vi "Enumerate Default Assert Strategies.vi"(11 "Banana":refnum<class "Banana.lvclass">) -> (1 "Strategies":T1, 3 "Banana":refnum<class "Banana.lvclass">)   [LabVIEW 2021, in "Bananas.lvlib" / "Platano.lvclass"]
uses:
  Platano.lvclass
  Banana/Banana.lvclass
  Assertion Strategies -- cluster.ctl
  AssertTrue/AssertTrue.lvclass
  AssertFalse/AssertFalse.lvclass
  AssertEqualValue/AssertEqualValue.lvclass
  AssertEqualType/AssertEqualType.lvclass
  AssertCompareValue/AssertCompareValue.lvclass
  AssetError/AssertError.lvclass
  AssertAlmostEqual/AssertAlmostEqualValue.lvclass
  Banana/Banana.lvclass/Banana.ctl
  <vilib>/LabVIEW Open Source Project/Data Manipulation/Variant/Variant_EmptyCluster.vi
  <vilib>/LabVIEW Open Source Project/Data Manipulation/TypeDescriptor/TypeDescriptor_SetName.vi
  <vilib>/Utility/GetType.llb/TD_Create Cluster.vi
  BananaPeel/BananaPeel.lvclass
  <vilib>/LabVIEW Open Source Project/Data Manipulation/Variant/OpenVariant.lvlib
  Bananas.lvlib
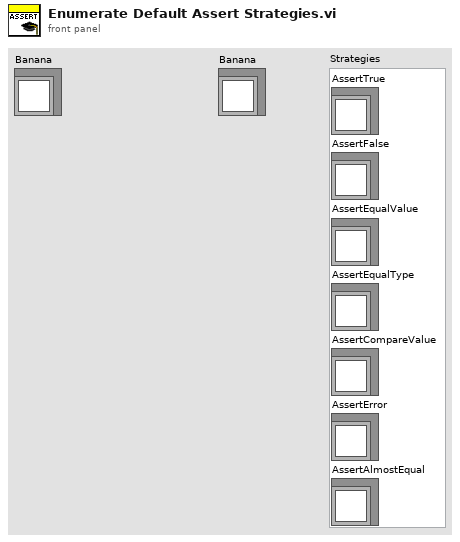
[diagram p1: front panel]
types:
  T1 = typedef "Bananas.lvlib/Assertion Strategies -- cluster.ctl" = cluster{"AssertTrue":refnum<class "AssertTrue.lvclass">, "AssertFalse":refnum<class "AssertFalse.lvclass">, "AssertEqualValue":refnum<class "AssertEqualValue.lvclass">, "AssertEqualType":refnum<class "AssertEqualType.lvclass">, "AssertCompareValue":refnum<class "AssertCompareValue.lvclass">, "AssertError":refnum<class "AssertError.lvclass">, "AssertAlmostEqual":refnum<class "AssertAlmostEqualValue.lvclass">}
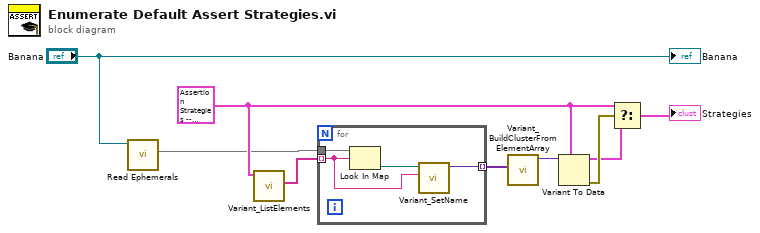
[diagram p0: block diagram]
diagram:
  w3 = T1 {"AssertTrue"=refnum, "AssertFalse"=refnum, "AssertEqualValue"=refnum, "AssertEqualType"=refnum, "AssertCompareValue"=refnum, "AssertError"=refnum, "AssertAlmostEqual"=refnum} ("Strategies")
  n1 = call "Read Ephemerals.vi"("Banana in"="Banana") -> ("Ephemerals"=w1:map{string, refnum<class "BananaPeel.lvclass">})  [unwired: 8 in, 2 out]
  n2 = call <vilib>:"Variant_ListElements.vi"("Variant"=w3) -> ("element names"=w9:string[])  [unwired: 7 in, 3 out]
  n3 = for {
    tunnel: w1 -> [w13]
    tunnel: w9 -> [w10] mode=indexing
    tunnel: [w11] -> w8 mode=indexing
    n4 = Look In Map(map=w13, key=w10) -> (value=w12:refnum<class "BananaPeel.lvclass">)  [unwired: 1 in, 1 out]
    n5 = call <vilib>:"Variant_SetName.vi"("Name"=w10, "Variant"=w12) -> ("Named Variant"=w11:variant)  [unwired: 9 in]
  }
  n6 = call <vilib>:"Variant_BuildClusterFromElementArray.vi"("Elements"=w8) -> ("Cluster"=w7:variant)  [unwired: 10 in]
  n7 = Variant To Data(type=w3, Variant=w7) -> (data=w5:T1, error out=w6:errorcluster)  [unwired: 1 in]
  n8 = Select(t=w3, s=w6, f=w5) -> (s? t:f=→"Strategies":T1)
  "Banana" <- "Banana"
